vi "Get All Structure Data.vi"(7 "Use Cached Data?":bool, 8 "Error In":errorcluster, 11 "Nest Config":T2) -> (0 "Error Out":errorcluster, 2 "Structures":T1[](array[typedef]), 3 "Nest Config":T2)   [LabVIEW 2013, in "LVH-Nest.lvlib"]
doc: "Read all data from all structures."
uses:
  LVH-Nest.lvlib
  Type Defs/Nest Config.ctl
  <vilib>/httpClient/ClientHandle.ctl
  Type Defs/Session Data.ctl
  Type Defs/Structure.ctl
  <vilib>/httpClient/LabVIEWHTTPClient.lvlib
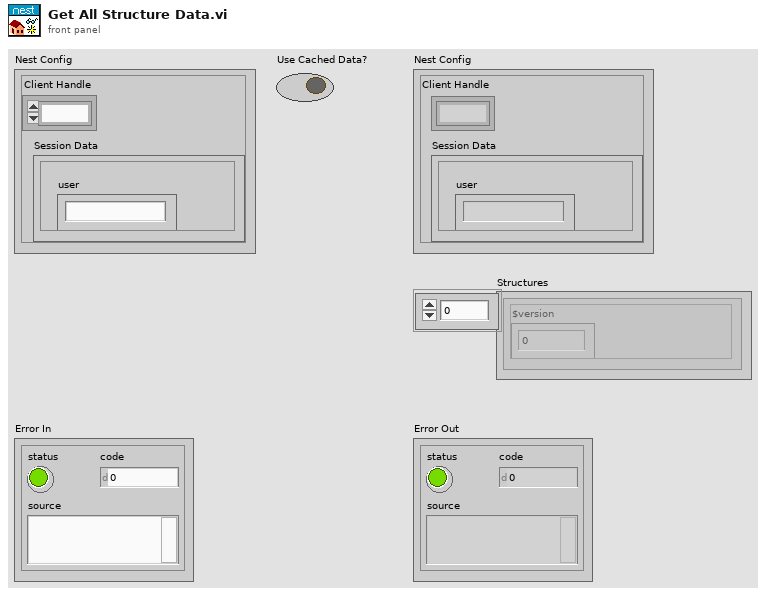
[diagram p1: front panel]
types:
  T1 = typedef "LVH-Nest.lvlib/Structure.ctl" = cluster{"$version":i32, "$timestamp":dbl, "dr_reminder_enabled":bool, "renovation_date":string, "country_code":string, "hvac_safety_shutoff_enabled":bool, "away":bool, "house_type":string, "topaz_enhanced_auto_away_enabled":bool, "name":string, "postal_code":string, "creation_time":dbl, "num_thermostats":string, "away_setter":dbl, "structure_area":dbl, "user":string, "devices":string[], "swarm":string[], "fabric_ids":string[]}
  T2 = typedef "LVH-Nest.lvlib/Nest Config.ctl" = cluster{"Client Handle":T3, "Session Data":T4}
  T3 = typedef "LabVIEWHTTPClient.lvlib/ClientHandle.ctl" = refnum<k1>
  T4 = typedef "LVH-Nest.lvlib/Session Data.ctl" = cluster{"is_superuser":bool, "is_staff":bool, "urls":cluster{"transport_url":string, "rubyapi_url":string, "weather_url":string, "log_upload_url":string, "support_url":string}, "limits":cluster{"thermostats_per_structure":u32, "structures":u32, "thermostats":u32, "smoke_detectors":u32, "smoke_detectors_per_structure":u32}, "access_token":string, "userid":string, "expires_in":string, "email":string, "user":string, "language":string}
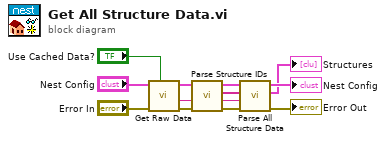
[diagram p0: block diagram]
diagram:
  n1 = call "Get Raw Data.vi"("Use Cached Data?"="Use Cached Data?", "Error In"="Error In", "Nest Config"="Nest Config") -> ("Error Out"=w11:errorcluster, "Data"=w10:string, "Nest Config"=w9:T2)  [unwired: 6 in]
  n2 = call "Parse Structure IDs.vi"("Error In"=w11, "Data"=w10, "Nest Config"=w9) -> ("Error Out"=w8:errorcluster, "Data"=w5:string, "Structure IDs"=w6:string[], "Nest Config"=w7:T2)  [unwired: 5 in]
  n3 = call "Parse All Structure Data.vi"("Error In"=w8, "Data"=w5, "Structure IDs"=w6, "Nest Config"=w7) -> ("Error Out"=→"Error Out":errorcluster, "Structures"=→"Structures":T1[], "Nest Config"=→"Nest Config":T2)  [unwired: 4 in, 1 out]
